vi "GetPose.vi"(9 "port":u16=22224, 10 "address":string="smlremote.no-ip.biz", 11 "QTM ID":i32) -> (3 "Pose":dbl[](array[numeric]))   [LabVIEW 2013]
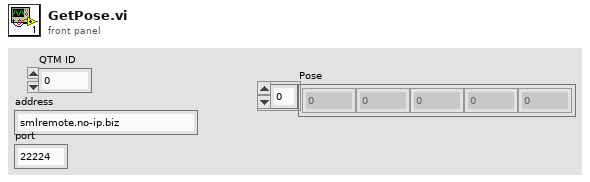
[diagram p1: front panel]
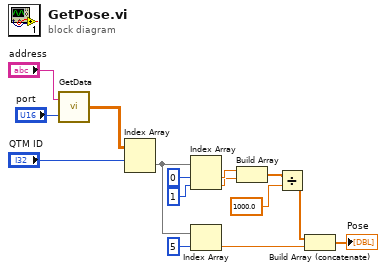
[diagram p0: block diagram]
diagram:
  n1 = call "GetData.vi"("port"="port", "address"="address") -> ("Poses"=w12:dbl[][])
  n2 = Index Array(array=w12, index (row)="QTM ID") -> (element=w8:dbl[])  [unwired: 1 in]
  n3 = Index Array(array=w8, index #1=0 ("index"), index #2=1 ("index")) -> (element #1=w3:dbl, element #2=w2:dbl)
  n4 = Index Array(array=w8, index=5) -> (element=w4:dbl)
  n5 = Build Array(w3, w2) -> (w1:dbl[])
  n6 = Divide(x=w1, y=1000.0) -> (x/y=w6:dbl[])
  n7 = Build Array (concatenate)(w6, w4) -> (→"Pose":dbl[])
